vi "high through put.vi"(7 "高通量？":bool, 10 "Array":T1[](array[typedef])) -> (2 "downSampling array":T1[](array[typedef]))   [LabVIEW 2017]
uses:
  <vilib>/vision/Image Controls.llb/IMAQ Image.ctl
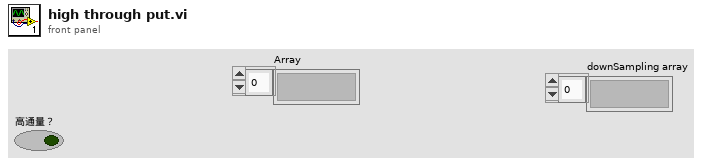
[diagram p1: front panel]
types:
  T1 = typedef "IMAQ Image.ctl" = refnum<image>
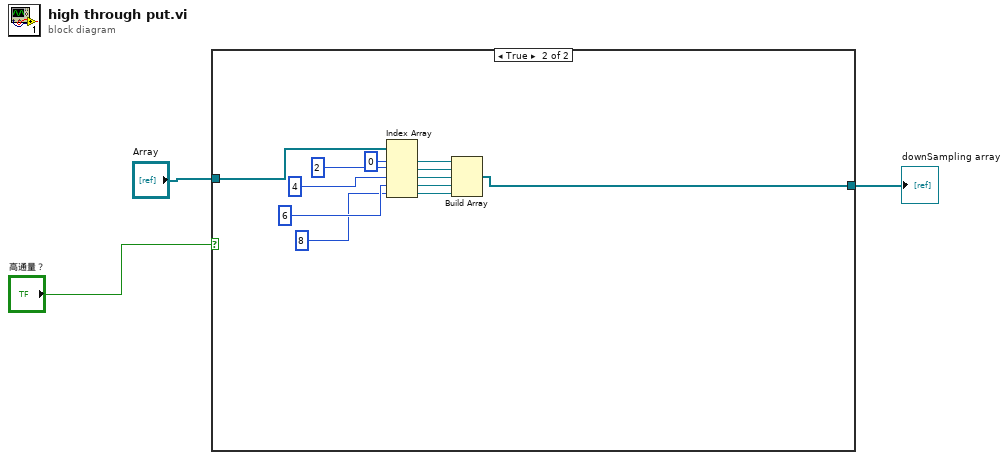
[diagram p0: block diagram]
diagram:
  n1 = case shown="True" "高通量？" {
    tunnel: "Array" -> [w4 w6]
    tunnel: [w4 w5] -> w2
    frame False {
    }
    frame True {
      n2 = Index Array(array=w6, index #1=0 ("index"), index #2=2 ("index"), index #3=4 ("index"), index #4=6 ("index"), index #5=8 ("index")) -> (element #1=w11:T1, element #2=w10:T1, element #3=w9:T1, element #4=w8:T1, element #5=w7:T1)
      n3 = Build Array(w11, w10, w9, w8, w7) -> (w5:T1[])
    }
  }
  "downSampling array" <- w2
